vi "Update Metadata channels.vi"(1 "Metadata Values":string[](array[string]), 2 "Metadata Names":string[](array[string]), 3 "Analysis info Cluster in":T1={"Colour"=0, "Inst type"=enum."Propeller anemometer", "Inst name"="", "Symbol"="", "Code name"="", "Extra Info"="", "Inst Array"=enum."PWA", "U"=0.0, "u^2"=0.0, "u^3"=0.0, "u^4"=0.0, "Skew_u"=0.0, "Kurt_u"=0.0, "Sd Error in Mean"=0.0, "% u'/U"=0.0, "X"=0.0, "Y"=0.0, "Z"=0.0, "Timescale integral Estimate"=0.0, "Sd Error in Variance"=0.0, "Calib File"=path "", "Calib Constants"=[], "Output Position"=FALSE, "Stats"=enum."None", "Av Sampling Rate"=0.0, "Av No of Samples"=0.0, "Total Meas Time (s)"=0.0, "OrigChName"="", "Max value"=0.0, "Min value"=0.0, "Req Sample Rate Hz"=0.0, "Sync Delay Time (s)"=0.0, "Ch No"=0, "Device"="", "Use Latest Calib"=FALSE, "Port"="", "Metadata Ch Names"=[], "Metadata Ch Values"=[], "Label"="", "chState"=enum."Solo", "Point Drift"=0.0, "inputConfig"=""} {"Kurt_u" format="%_3g"; "u^4" format="%_3g"; "u^3" format="%_3g"; "Sd Error in Variance" format="%_3g"; "u^2" format="%_3g"; "Sd Error in Mean" format="%_3g"; "U" format="%_3g"; "Sync Delay Time (s)" format="%.4f"; "Total Meas Time (s)" format="%_5g"; "Skew_u" format="%_3g"; "% u'/U" format="%_3g"}) -> (0 "Analysis info Cluster out":T1={"Colour"=0, "Inst type"=enum."Propeller anemometer", "Inst name"="", "Symbol"="", "Code name"="", "Extra Info"="", "Inst Array"=enum."PWA", "U"=0.0, "u^2"=0.0, "u^3"=0.0, "u^4"=0.0, "Skew_u"=0.0, "Kurt_u"=0.0, "Sd Error in Mean"=0.0, "% u'/U"=0.0, "X"=0.0, "Y"=0.0, "Z"=0.0, "Timescale integral Estimate"=0.0, "Sd Error in Variance"=0.0, "Calib File"=path "", "Calib Constants"=[], "Output Position"=FALSE, "Stats"=enum."None", "Av Sampling Rate"=0.0, "Av No of Samples"=0.0, "Total Meas Time (s)"=0.0, "OrigChName"="", "Max value"=0.0, "Min value"=0.0, "Req Sample Rate Hz"=0.0, "Sync Delay Time (s)"=0.0, "Ch No"=0, "Device"="", "Use Latest Calib"=FALSE, "Port"="", "Metadata Ch Names"=[], "Metadata Ch Values"=[], "Label"="", "chState"=enum."Solo", "Point Drift"=0.0, "inputConfig"=""} {"Kurt_u" format="%_3g"; "u^4" format="%_3g"; "u^3" format="%_3g"; "Sd Error in Variance" format="%_3g"; "u^2" format="%_3g"; "Sd Error in Mean" format="%_3g"; "U" format="%_3g"; "Sync Delay Time (s)" format="%.4f"; "Total Meas Time (s)" format="%_5g"; "Skew_u" format="%_3g"; "% u'/U" format="%_3g"})   [LabVIEW 2022 SP3]
uses:
  Controls/Inst_type.ctl
  Controls/Instrument_Array.ctl
  Controls/Analysis_info_cluster.ctl
  Controls/channelState.ctl
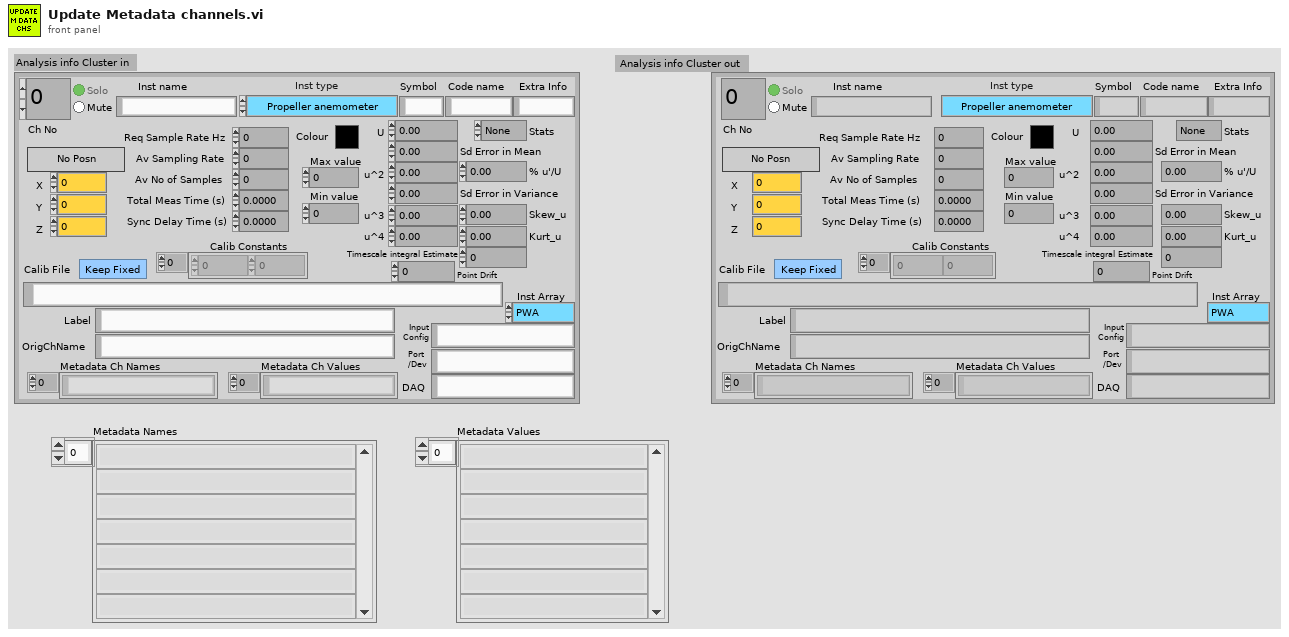
[diagram p1: front panel]
types:
  T1 = typedef "Analysis_info_cluster.ctl" = cluster{"Colour":u32, "Inst type":T2, "Inst name":string, "Symbol":string, "Code name":string, "Extra Info":string, "Inst Array":T3, "U":dbl, "u^2":dbl, "u^3":dbl, "u^4":dbl, "Skew_u":dbl, "Kurt_u":dbl, "Sd Error in Mean":dbl, "% u'/U":dbl, "X":dbl, "Y":dbl, "Z":dbl, "Timescale integral Estimate":dbl, "Sd Error in Variance":dbl, "Calib File":path, "Calib Constants":dbl[], "Output Position":bool, "Stats":enum16{"None", "Basic", "Full"}, "Av Sampling Rate":dbl, "Av No of Samples":dbl, "Total Meas Time (s)":dbl, "OrigChName":string, "Max value":dbl, "Min value":dbl, "Req Sample Rate Hz":dbl, "Sync Delay Time (s)":dbl, "Ch No":i16, "Device":string, "Use Latest Calib":bool, "Port":string, "Metadata Ch Names":string[], "Metadata Ch Values":string[], "Label":string, "chState":T4, "Point Drift":dbl, "inputConfig":string}
  T2 = typedef "Inst_type.ctl" = enum16{"Raw voltage", "Raw with zero offsetting", "Propeller anemometer", "Pressure Transducer", "Pitot-static tube", "Hot wire", "Cross wire 1", "Cross wire 2", "Generic Linear", "Generic Polynomial", "Generic BackPoly", "Fast FID", "Thermocouple", "Cold wire", "Pulsed Wire", "LDA Vel", "LDA Tran time", "LDA Arr time", "Microphone"}
  T3 = typedef "Instrument_Array.ctl" = enum16{"PWA", "LDA", "Analogue"}
  T4 = typedef "channelState.ctl" = enum32{"No Selection", "Solo", "Mute"}
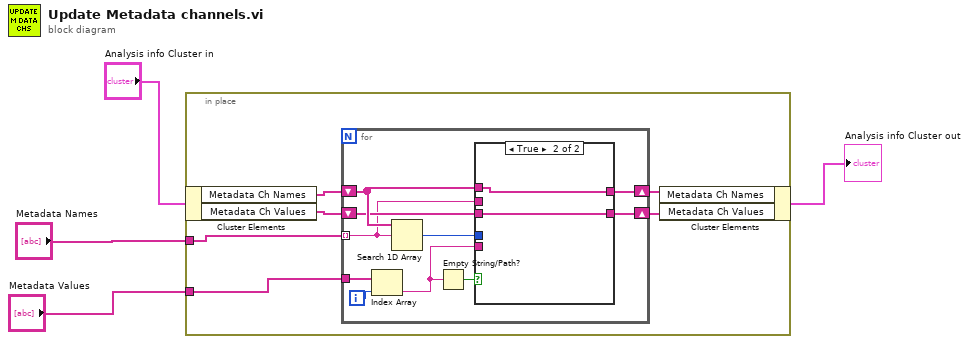
[diagram p0: block diagram]
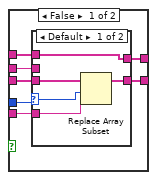
[diagram p2: hidden frame]
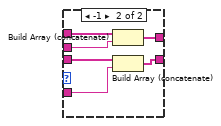
[diagram p3: hidden frame]
diagram:
  n1 = in-place {
    in-place-border: "Metadata Names" -> [w10]
    in-place-border: "Metadata Values" -> [w5]
    n2 = in-place-cluster #1("Analysis info Cluster in") -> ("Metadata Ch Names"=w9:string[], "Metadata Ch Values"=w7:string[])
    n3 = for {
      tunnel: w10 -> [w15] mode=indexing
      shift-right: [w19] -> w8
      shift-left: w9 -> [w18]
      shift-right: [w16] -> w6
      shift-left: w7 -> [w17]
      tunnel: w5 -> [w13]
      i -> [w12]
      n4 = Index Array(array=w13, index=w12) -> (element=w11:string)
      n5 = Search 1D Array(1D array=w18, element=w15) -> (index of element=w20:i32)  [unwired: 1 in]
      n6 = Empty String/Path?(string/path=w11) -> (empty?=w14:bool)
      n7 = case shown="True" w14 {
        tunnel: w20 -> [w27 _]
        tunnel: [w26 w40] -> w19
        tunnel: w18 -> [w25 w40]
        tunnel: w17 -> [w24 w39]
        tunnel: [w23 w39] -> w16
        tunnel: w15 -> [w22 _]
        tunnel: w11 -> [w21 _]
        frame False {
          n8 = case shown="Default" w27 {
            selector: w27 -> [w29 _]
            tunnel: w25 -> [w32 w38]
            tunnel: [w32 w37] -> w26
            tunnel: w22 -> [_ w36]
            tunnel: w21 -> [w28 w35]
            tunnel: w24 -> [w31 w34]
            tunnel: [w30 w33] -> w23
            frame Default {
              n9 = Replace Array Subset(array=w31, new element=w28, index=w29) -> (w30:string[])
            }
            frame -1 {
              n10 = Build Array (concatenate)(w38, w36) -> (w37:string[])
              n11 = Build Array (concatenate)(w34, w35) -> (w33:string[])
            }
          }
        }
        frame True {
        }
      }
    }
    n12 = in-place-cluster #1("Metadata Ch Names"=w8, "Metadata Ch Values"=w6) -> (→"Analysis info Cluster out":T1)
  }
